vi "Configure Air to DUT max temperature difference.vi"(8 "error in (no error)":errorcluster, 9 "Air to DUT Max Temperature Difference (300)":dbl=300.0 min=10.0 max=300.0 step=1.0, 11 "VISA resource name":refnum<visa-resource-name>) -> (0 "error out":errorcluster, 3 "VISA resource name out":refnum<visa-resource-name>)   [LabVIEW 2012, in "Temptronic TP04300.lvlib"]
doc: "This VI configures a maximum air to DUT temperature difference for TP04300 instrument.\n\n<b>Air to DUT MAX Temperature Difference</b> configures the maximum allowable air to DUT temperature difference in Celsius for both air and DUT modes \nin 1 degree increments.\n\nDefault Value: 300.0\nValid Range: 1.0 - 300.0"
uses:
  <instrlib>/Temptronic TP04300/Temptronic TP04300.lvlib
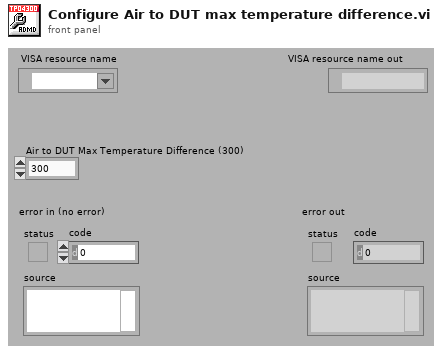
[diagram p1: front panel]
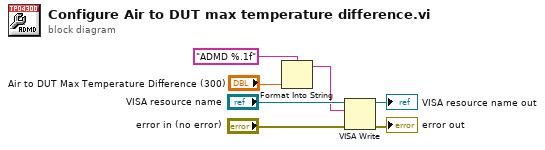
[diagram p0: block diagram]
diagram:
  n1 = Format Into String(format string="ADMD %.1f" ("multi-line string"), "Air to DUT Max Temperature Difference (300)") -> (resulting string=w3:string)  [unwired: 2 in, 1 out]
  n2 = VISA Write(VISA resource name="VISA resource name", write buffer=w3, error in (no error)="error in (no error)") -> (VISA resource name out=→"VISA resource name out":refnum<visa-resource-name>, error out=→"error out":errorcluster)  [unwired: 1 out]
